vi "Get SMO.vi"(8 "error in (no error)":errorcluster, 11 "SMO.UI":refnum<class "SMO.UI.Template.lvclass">) -> (0 "error out":errorcluster, 2 "SMO.Template":refnum<class "SMO.Template.lvclass">, 3 "SMO.UI out":refnum<class "SMO.UI.Template.lvclass">)   [LabVIEW 2013, in "SMO.UI.Template.lvclass"]
doc: "Gets the SMO dependency."
uses:
  SMO.UI.Template.lvclass
  SMO.Template/SMO.Template.lvclass
  SMO.UI.Template.lvclass/SMO.UI.Template.ctl
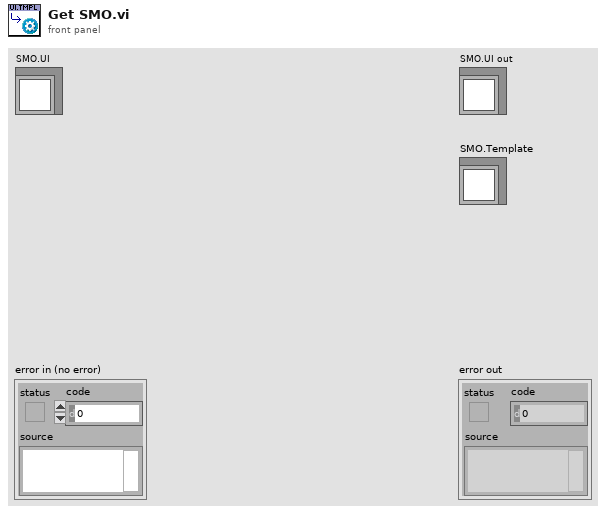
[diagram p1: front panel]
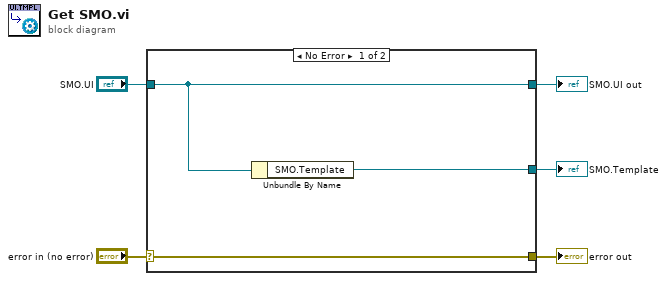
[diagram p0: block diagram]
diagram:
  n1 = case shown="No Error" "error in (no error)" {
    selector: "error in (no error)" -> [w8 w9]
    tunnel: [w8 w9] -> w4
    tunnel: [w7 w10] -> w2
    tunnel: "SMO.UI" -> [w7 w10]
    tunnel: [w6 _] -> w1
    frame No Error {
      n2 = Unbundle By Name(w7) -> ("SMO.Template"=w6:refnum<class "SMO.Template.lvclass">)
    }
    frame Error {
    }
  }
  "error out" <- w4
  "SMO.UI out" <- w2
  "SMO.Template" <- w1
